vi "Finish.vi"   [LabVIEW 2012]
doc: "This VI is called just before exiting. It is expected to close I/O refnum, save collected data, etc."
uses:
  <vilib>/Rock Robotics/WPI/Joystick/WPI_JoystickGetSetRefNum.vi
  <vilib>/Rock Robotics/WPI/Compressor/WPI_CompressorGetSetRefNum.vi
  <vilib>/Rock Robotics/WPI/RobotDrive/WPI_RobotDriveGetSetRefNum.vi
types:
  T1 = typedef "WPI_MotorControlDeviceRef.ctl" = cluster{"DeviceStatus":errorcluster, "Type":enum16{"PWM", "CAN"}, "PWM":cluster{"Digital Module":T2, "PWM Channel":T3, "DeadBand":T4}, "CAN":cluster{"Device Number":u8, "Control Mode":T5, "Semaphore":T6, "Max Vout":dbl}, "Invert":bool, "TransformRef":T7, "InvTransformRef":T7}
  T2 = typedef "FPGA_TypedefDigitalModule.ctl" = enum16{"Digital Module 1", "Digital Module 2"}
  T3 = typedef "FPGA_DIOPWMChannel.ctl" = enum8{"PWM 1", "PWM 2", "PWM 3", "PWM 4", "PWM 5", "PWM 6", "PWM 7", "PWM 8", "PWM 9", "PWM 10", "Invalid"}
  T4 = typedef "WPI_PWMDeadband.ctl" = cluster{"Name":string, "maxPositivePwm":i32, "minPositivePwm":i32, "centerPwm":i32, "maxNegativePwm":i32, "minNegativePwm":i32, "angularRange":u16}
  T5 = typedef "WPI_CANJaguar_ControlMode.ctl" = enum8{"Percent VBus", "Current", "Speed", "Position", "Voltage"}
  T6 = typedef "Semaphore RefNum" = refnum<k1>
  T7 = typedef "WPI_PWMTransform_ConPane.ctl" = refnum<vi>
  T8 = typedef "WPI_JoystickDevRef.ctl" = cluster{"Device":T9}
  T9 = typedef "WPI_JoystickDeviceEnum.ctl" = enum16{"USB 1", "USB 2", "USB 3", "USB 4", "Kinect 1", "Kinect 2"}
  T10 = typedef "WPI_RobotDriveDevRef.ctl" = cluster{"DevStatus":errorcluster, "Motors[]":T1[], "Square Inputs":bool, "Max Output":dbl, "Isochronous":bool}
  T11 = typedef "WPI_RelayDevRef.ctl" = cluster{"DevStatus":errorcluster, "Relay Channel":T12, "Digital Module":T2, "Relay Direction":T13}
  T12 = typedef "FPGA_DIORelayChannel.ctl" = enum8{"Relay 1", "Relay 2", "Relay 3", "Relay 4", "Relay 5", "Relay 6", "Relay 7", "Relay 8", "Invalid"}
  T13 = typedef "WPI_RelayDirection.ctl" = enum16{"Both directions", "Forward only", "Reverse only"}
  T14 = typedef "WPI_CameraDevRef.ctl" = cluster{"Camera Address":string, "CameraStatus":errorcluster, "Acquire Image Notifier":refnum<notifier>}
  T15 = typedef "WPI_CompressorDevRef.ctl" = cluster{"DevStatus":errorcluster, "DigitalInputDevRef":T16, "RelayDevRef":T11}
  T16 = typedef "WPI_DigitalInputDevRef.ctl" = cluster{"DevStatus":errorcluster, "DIO Channel":T17, "Digital Module":T2}
  T17 = typedef "FPGA_DIOChannel.ctl" = enum8{"DIO 1", "DIO 2", "DIO 3", "DIO 4", "DIO 5", "DIO 6", "DIO 7", "DIO 8", "DIO 9", "DIO 10", "DIO 11", "DIO 12", "DIO 13", "DIO 14", "Invalid"}
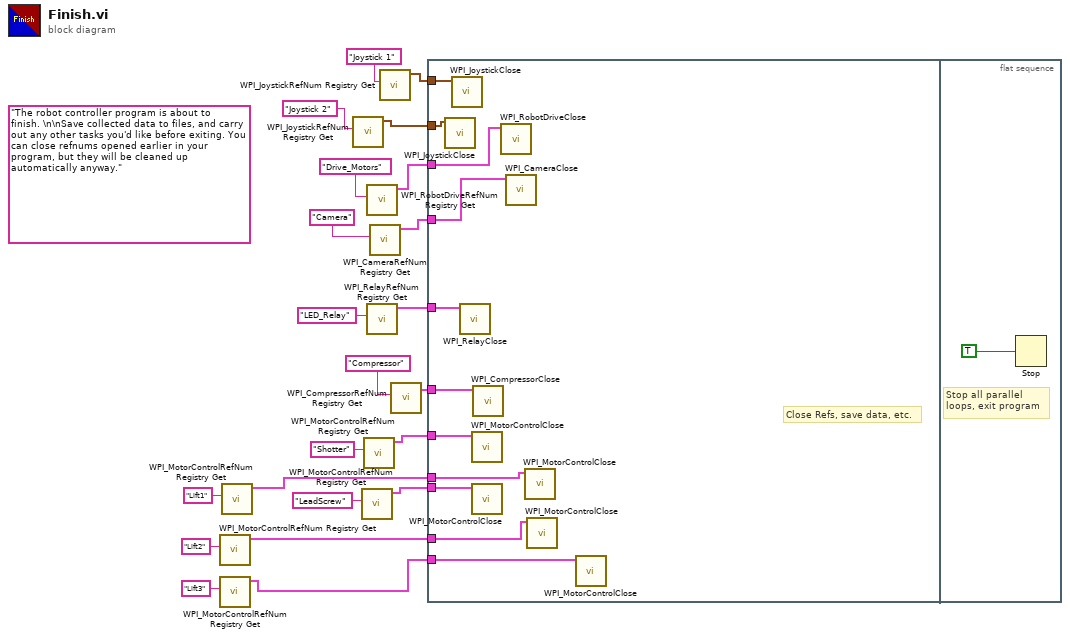
[diagram p0: block diagram]
diagram:
  (unwired) "The robot controller program is about to finish. \n\nSave collected data to files, and carry out any other tasks you'd like before exiting. You can close refnums opened earlier in your program, but they will be cleaned up automatically anyway."
  n1 = call <vilib>:"WPI_MotorControlRefNum Registry Get.vi"("refnum name"="Lift2") -> ("MotorControlDevRef"=w2:T1)  [unwired: 9 in, 1 out]
  n2 = call <vilib>:"WPI_MotorControlRefNum Registry Get.vi"("refnum name"="Lift3") -> ("MotorControlDevRef"=w1:T1)  [unwired: 9 in, 1 out]
  n3 = call <vilib>:"WPI_MotorControlRefNum Registry Get.vi"("refnum name"="Lift1") -> ("MotorControlDevRef"=w3:T1)  [unwired: 9 in, 1 out]
  n4 = call <vilib>:"WPI_JoystickRefNum Registry Get.vi"("refnum name"="Joystick 2") -> ("JoystickDevRef"=w8:T8)  [unwired: 1 in, 9 out]
  n5 = call <vilib>:"WPI_MotorControlRefNum Registry Get.vi"("refnum name"="LeadScrew") -> ("MotorControlDevRef"=w9:T1)  [unwired: 9 in, 1 out]
  n6 = call <vilib>:"WPI_MotorControlRefNum Registry Get.vi"("refnum name"="Shotter") -> ("MotorControlDevRef"=w11:T1)  [unwired: 9 in, 1 out]
  n7 = call <vilib>:"WPI_RobotDriveRefNum Registry Get.vi"("refnum name"="Drive_Motors") -> ("RobotDriveDevRef"=w20:T10)  [unwired: 1 in, 9 out]
  n8 = call <vilib>:"WPI_RelayRefNum Registry Get.vi"("refnum name"="LED_Relay") -> ("RelayDevRef"=w13:T11)  [unwired: 9 in, 1 out]
  n9 = call <vilib>:"WPI_CameraRefNum Registry Get.vi"("refnum name"="Camera") -> ("CameraDevRef"=w18:T14)  [unwired: 1 in, 9 out]
  n10 = call <vilib>:"WPI_JoystickRefNum Registry Get.vi"("refnum name"="Joystick 1") -> ("JoystickDevRef"=w19:T8)  [unwired: 1 in, 9 out]
  n11 = call <vilib>:"WPI_CompressorRefNum Registry Get.vi"("refnum name"="Compressor") -> ("CompressorDevRef"=w15:T15)  [unwired: 9 in, 1 out]
  n12 = flat-sequence {
    tunnel: w20 -> [w33]
    tunnel: w19 -> [w32]
    tunnel: w18 -> [w31]
    tunnel: w15 -> [w30]
    tunnel: w13 -> [w29]
    tunnel: w11 -> [w28]
    tunnel: w9 -> [w27]
    tunnel: w8 -> [w26]
    tunnel: w3 -> [w25]
    tunnel: w2 -> [w24]
    tunnel: w1 -> [w23]
    frame #0 {
      # "Close Refs, save data, etc."
      n13 = call <vilib>:"WPI_JoystickClose.vi"("JoystickDevRef"=w26) -> ()  [unwired: 11 out]
      n14 = call <vilib>:"WPI_JoystickClose.vi"("JoystickDevRef"=w32) -> ()  [unwired: 11 out]
      n15 = call <vilib>:"WPI_RelayClose.vi"("RelayDevRef"=w29) -> ()  [unwired: 10 in, 1 out]
      n16 = call <vilib>:"WPI_MotorControlClose.vi"("MotorControlDevRef"=w28) -> ()  [unwired: 10 in, 1 out]
      n17 = call <vilib>:"WPI_MotorControlClose.vi"("MotorControlDevRef"=w27) -> ()  [unwired: 10 in, 1 out]
      n18 = call <vilib>:"WPI_CompressorClose.vi"("CompressorDevRef"=w30) -> ()  [unwired: 10 in, 1 out]
      n19 = call <vilib>:"WPI_RobotDriveClose.vi"("RobotDriveDevRef"=w33) -> ()  [unwired: 1 in, 10 out]
      n20 = call <vilib>:"WPI_CameraClose.vi"("CameraDevRef"=w31) -> ()  [unwired: 1 in, 10 out]
      n21 = call <vilib>:"WPI_MotorControlClose.vi"("MotorControlDevRef"=w25) -> ()  [unwired: 10 in, 1 out]
      n22 = call <vilib>:"WPI_MotorControlClose.vi"("MotorControlDevRef"=w24) -> ()  [unwired: 10 in, 1 out]
      n23 = call <vilib>:"WPI_MotorControlClose.vi"("MotorControlDevRef"=w23) -> ()  [unwired: 10 in, 1 out]
    }
    frame #1 {
      # "Stop all parallel\nloops, exit program"
      n24 = Stop(stop? (T)=TRUE ("Quit")) -> ()
    }
  }
